vi "_Update Parameter Data.vi"(4 "error in":errorcluster, 7 "Parameter":T1 {"Expt"."Mass Range"."Resolution Type" items=["High/High", "Medium/Medium", "Low/Low", "High/Medium", "High/Low", "Medium/High", "Medium/Low", "Low/High", "Low/Medium"]}) -> (0 "error out":errorcluster, 1 "Last memory index":u16, 3 "RF Only":bool)   [LabVIEW 2015]
uses:
  Type/_RT Parameter.ctl
  Type/_RT Active Ch.ctl
  Type/_RT Expt.ctl
  Type/_Run Mode.ctl
  Type/_RT Mass Range.ctl
  Type/_RT Res Type.ctl
  _RT Global.vi
  <vilib>/Utility/error.llb/Error Cluster From Error Code.vi
  <vilib>/rvi/errors/niLvFpgaAdjustHostInterfaceError.vi
  <vilib>/rvi/interface/nirviReadWriteControl/nirviReadWriteControl.xnode
  Type/FPGA Typedef.ctl
  FPGA Bitfiles/FPGA9607.lvbitx
  NiFpgaLv.dll
panel:
  out "x-y":u32
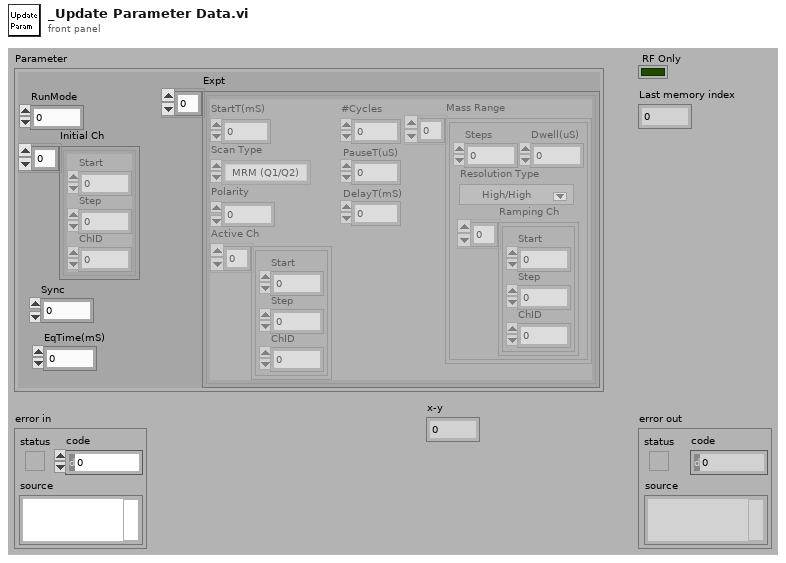
[diagram p1: front panel]
types:
  T1 = typedef "_RT Parameter.ctl" = cluster{"RunMode":i32, "Initial Ch":T2[], "Sync":u8, "Expt":T3[], "EqTime(mS)":i32}
  T2 = typedef "_RT Active Ch.ctl" = cluster{"Start":i32, "Step":i32, "ChID":i32}
  T3 = typedef "_RT Expt.ctl" = cluster{"StartT(mS)":i32, "#Cycles":i32, "Scan Type":T4, "PauseT(uS)":i32, "Polarity":u8, "DelayT(mS)":i32, "Active Ch":T2[], "Mass Range":T5[]}
  T4 = typedef "_Run Mode.ctl" = enum16{"MRM (Q1/Q2)", "Q1 Scan", "Q1 SRM", "Q2 Scan", "Q2 SRM", "Product Scan", "Precursor Scan", "Neutral Loss", "Neutral Gain"}
  T5 = typedef "_RT Mass Range.ctl" = cluster{"Steps":i32, "Dwell(uS)":i32, "Resolution Type":T6, "Ramping Ch":T2[]}
  T6 = typedef "_RT Res Type.ctl" = u16
  T7 = typedef "FPGA Typedef.ctl" = refnum<k20>
  T8 = typedef "_RT Configuration 2.ctl" = cluster{"Name":string, "Ch#":u8, "Min":dbl, "Max":dbl, "Def+":dbl, "Def-":dbl, "Offset":dbl, "Slope":dbl, "Type":u8, "Description":string, "SettleT":dbl}
  T9 = typedef "_RT Instrument 2.ctl" = cluster{"Table":T8[], "Instrument":string[]}
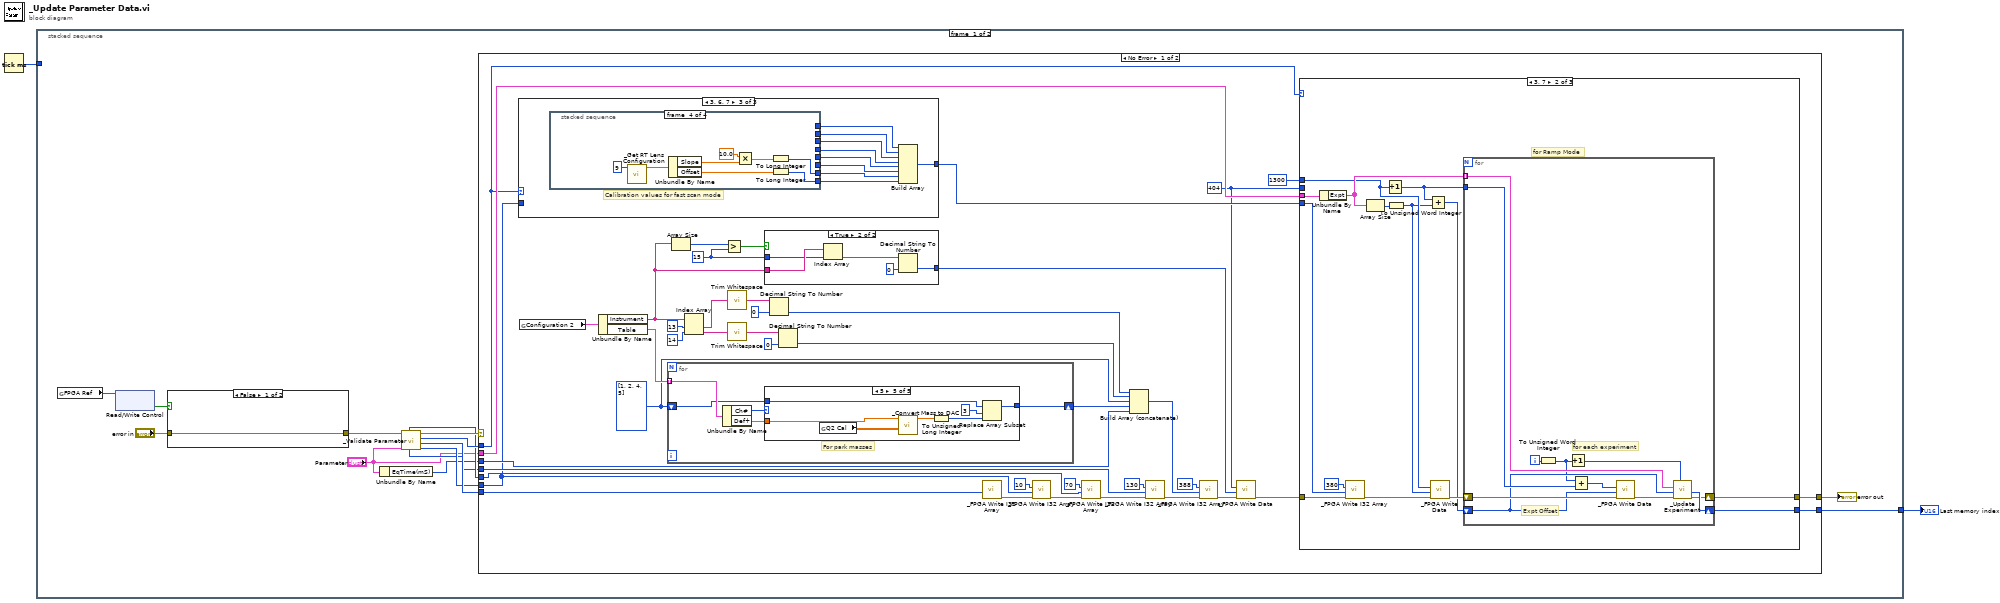
[diagram p0: block diagram]
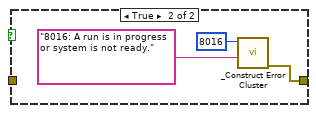
[diagram p2: hidden frame]
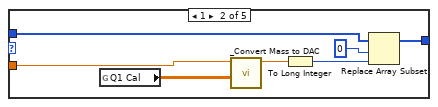
[diagram p5: hidden frame]
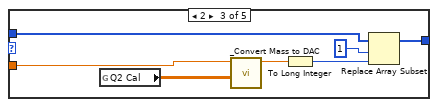
[diagram p6: hidden frame]
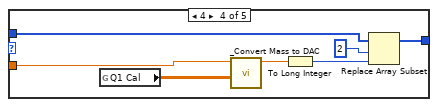
[diagram p7: hidden frame]
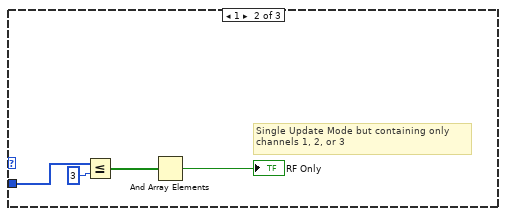
[diagram p9: hidden frame]
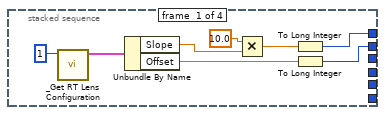
[diagram p10: hidden frame]
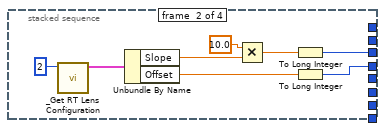
[diagram p11: hidden frame]
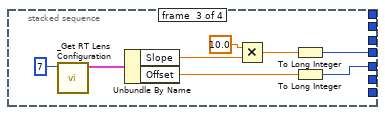
[diagram p12: hidden frame]
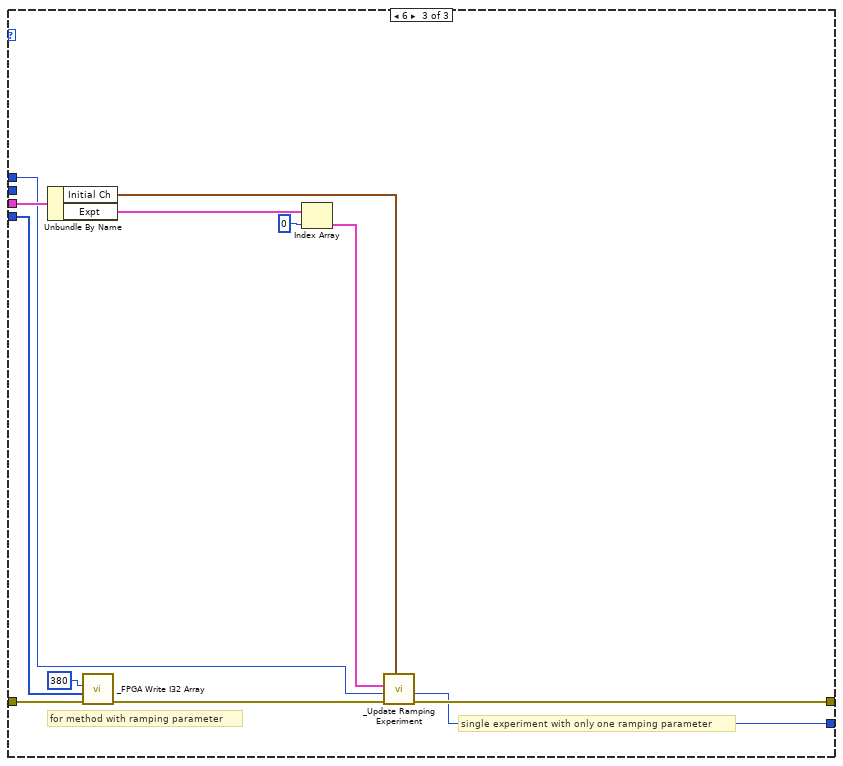
[diagram p14: hidden frame]
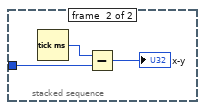
[diagram p16: hidden frame]
diagram:
  n1 = Tick Count (ms)() -> (millisecond timer value=w2:u32)
  n2 = stacked-sequence {
    tunnel: w2 -> [_ w189]
    tunnel: [w3 _] -> w1
    frame #0 {
      n3 = global read "_RT Global.vi" "FPGA Ref"() -> (w4:T7)
      n4 = xnode "Read/Write Control"("FPGA VI Reference In"=w4) -> ("Running"=w7:bool)  [unwired: 1 in, 2 out]
      n5 = case shown="False" w7 {
        tunnel: [w17 w18] -> w6
        tunnel: "error in" -> [w17 _]
        frame False {
        }
        frame True {
          n6 = call "_Construct Error Cluster.vi"("reason"="8016: A run is in progress or system is not ready.", "errorCode"=8016) -> ("error out"=w18:errorcluster)  [unwired: 2 in, 3 out]
        }
      }
      n7 = Unbundle By Name("Parameter") -> ("EqTime(mS)"=w8:i32)
      n8 = call "_Validate Parameter.vi"("Parameter"="Parameter", "error in (no error)"=w6) -> ("Ch ID"=w12:i32[], "General Param"=w13:i32[], "RunMode"=w14:i32, "error out"=w15:errorcluster, "Low Values"=w10:i32[], "High Values (DAC)"=w11:i32[])  [unwired: 2 out]
      n9 = case shown="No Error" w15 {
        selector: w15 -> [_ w187]
        tunnel: [w62 w187] -> w16
        tunnel: w14 -> [w50 _]
        tunnel: w13 -> [w60 _]
        tunnel: w12 -> [w31 _]
        tunnel: w11 -> [w55 _]
        tunnel: w10 -> [w53 _]
        tunnel: "Parameter" -> [w61 _]
        tunnel: w8 -> [w34 _]
        tunnel: [w23 _] -> w3
        frame No Error {
          w25 = 15 ("y")
          w22 = u16 404 ("y")
          w36 = u32[] [1, 2, 4, 5]
          n10 = case shown="3, 6, 7" w50 {
            tunnel: [_ _ w107] -> w49
            tunnel: w31 -> [_ w106 _]
            frame 0, Default {
            }
            frame 1 {
              # "Single Update Mode but containing only\nchannels 1, 2, or 3"
              n11 = Less Or Equal?(x=w106, y=3) -> (x <= y?=w104:bool[])
              n12 = And Array Elements(Boolean array=w104) -> (logical AND=→"RF Only":bool)
            }
            frame 3, 6, 7 {
              # "Calibration values for fast scan mode"
              n13 = stacked-sequence {
                tunnel: [w117 _ _ _] -> w108
                tunnel: [w116 _ _ _] -> w109
                tunnel: [_ w125 _ _] -> w110
                tunnel: [_ w124 _ _] -> w111
                tunnel: [_ _ w133 _] -> w112
                tunnel: [_ _ w132 _] -> w113
                tunnel: [_ _ _ w141] -> w114
                tunnel: [_ _ _ w140] -> w115
                frame #0 {
                  n14 = call "_Get RT Lens Configuration.vi"("Channel #"=u8 1) -> ("Lens Configuration"=w122:T8)  [unwired: 1 in, 5 out]
                  n15 = Unbundle By Name(w122) -> ("Slope"=w120:dbl, "Offset"=w121:dbl)
                  n16 = Multiply(x=10.0, y=w120) -> (x*y=w118:dbl)
                  n17 = To Long Integer(number=w118) -> (32bit integer=w117:i32)
                  n18 = To Long Integer(number=w121) -> (32bit integer=w116:i32)
                }
                frame #1 {
                  n19 = call "_Get RT Lens Configuration.vi"("Channel #"=u8 2) -> ("Lens Configuration"=w130:T8)  [unwired: 1 in, 5 out]
                  n20 = Unbundle By Name(w130) -> ("Slope"=w128:dbl, "Offset"=w129:dbl)
                  n21 = Multiply(x=10.0, y=w128) -> (x*y=w126:dbl)
                  n22 = To Long Integer(number=w126) -> (32bit integer=w125:i32)
                  n23 = To Long Integer(number=w129) -> (32bit integer=w124:i32)
                }
                frame #2 {
                  n24 = call "_Get RT Lens Configuration.vi"("Channel #"=u8 7) -> ("Lens Configuration"=w138:T8)  [unwired: 1 in, 5 out]
                  n25 = Unbundle By Name(w138) -> ("Slope"=w136:dbl, "Offset"=w137:dbl)
                  n26 = Multiply(x=10.0, y=w136) -> (x*y=w134:dbl)
                  n27 = To Long Integer(number=w134) -> (32bit integer=w133:i32)
                  n28 = To Long Integer(number=w137) -> (32bit integer=w132:i32)
                }
                frame #3 {
                  n29 = call "_Get RT Lens Configuration.vi"("Channel #"=u8 9) -> ("Lens Configuration"=w146:T8)  [unwired: 1 in, 5 out]
                  n30 = Unbundle By Name(w146) -> ("Slope"=w144:dbl, "Offset"=w145:dbl)
                  n31 = Multiply(x=10.0, y=w144) -> (x*y=w142:dbl)
                  n32 = To Long Integer(number=w142) -> (32bit integer=w141:i32)
                  n33 = To Long Integer(number=w145) -> (32bit integer=w140:i32)
                }
              }
              n34 = Build Array(w108, w109, w110, w111, w112, w113, w114, w115) -> (w107:i32[])
            }
          }
          n35 = global read "_RT Global.vi" "Configuration 2"() -> (w48:T9)
          n36 = Unbundle By Name(w48) -> ("Instrument"=w26:string[], "Table"=w41:T8[])
          n37 = for {
            tunnel: w41 -> [w73] mode=indexing
            shift-right: [w70] -> w35
            shift-left: w36 -> [w71]
            # "For park masses"
            n38 = Unbundle By Name(w73) -> ("Ch#"=w72:u8, "Def+"=w69:dbl)
            n39 = case shown="5" w72 {
              tunnel: w71 -> [w74 w78 w85 w92 w99]
              tunnel: [w74 w75 w82 w89 w96] -> w70
              tunnel: w69 -> [_ w81 w88 w95 w102]
              frame 0, Default {
              }
              frame 1 {
                n40 = global read "_RT Global.vi" "Q1 Cal"() -> (w80:dbl[][])
                n41 = call "_Convert Mass to DAC.vi"("Calibration Table"=w80, "Mass"=w81) -> ("DAC Value"=w79:dbl)  [unwired: 2 in, 3 out]
                n42 = To Long Integer(number=w79) -> (32bit integer=w76:i32)
                n43 = Replace Array Subset(array=w78, new element=w76, index=0) -> (w75:u32[])
              }
              frame 2 {
                n44 = global read "_RT Global.vi" "Q2 Cal"() -> (w87:dbl[][])
                n45 = call "_Convert Mass to DAC.vi"("Calibration Table"=w87, "Mass"=w88) -> ("DAC Value"=w86:dbl)  [unwired: 2 in, 3 out]
                n46 = To Long Integer(number=w86) -> (32bit integer=w83:i32)
                n47 = Replace Array Subset(array=w85, new element=w83, index=1) -> (w82:u32[])
              }
              frame 4 {
                n48 = global read "_RT Global.vi" "Q1 Cal"() -> (w94:dbl[][])
                n49 = call "_Convert Mass to DAC.vi"("Calibration Table"=w94, "Mass"=w95) -> ("DAC Value"=w93:dbl)  [unwired: 2 in, 3 out]
                n50 = To Long Integer(number=w93) -> (32bit integer=w90:i32)
                n51 = Replace Array Subset(array=w92, new element=w90, index=2) -> (w89:u32[])
              }
              frame 5 {
                n52 = global read "_RT Global.vi" "Q2 Cal"() -> (w101:dbl[][])
                n53 = call "_Convert Mass to DAC.vi"("Calibration Table"=w101, "Mass"=w102) -> ("DAC Value"=w100:dbl)  [unwired: 2 in, 3 out]
                n54 = To Unsigned Long Integer(number=w100) -> (unsigned 32bit integer=w97:u32)
                n55 = Replace Array Subset(array=w99, new element=w97, index=3) -> (w96:u32[])
              }
            }
          }
          n56 = Array Size(array=w26) -> (size(s)=w28:i32)
          n57 = Index Array(array=w26, index #1=13 ("index"), index #2=14 ("index")) -> (element #1=w45:string, element #2=w44:string)
          n58 = Greater?(x=w28, y=w25) -> (0:w27:bool)
          n59 = call <vilib>:"Trim Whitespace.vi"("string"=w45) -> ("trimmed string"=w33:string)  [unwired: 1 in]
          n60 = call <vilib>:"Trim Whitespace.vi"("string"=w44) -> ("trimmed string"=w43:string)  [unwired: 1 in]
          n61 = case shown="True" w27 {
            tunnel: w26 -> [_ w68]
            tunnel: w25 -> [w63 w66]
            tunnel: [w63 w65] -> w24
            frame False {
            }
            frame True {
              n62 = Index Array(array=w68, index=w66) -> (element=w67:string)
              n63 = Decimal String To Number(string=w67, default (0L)=u32 0 ("default (0 I32)")) -> (number=w65:u32)  [unwired: 2 out]
            }
          }
          n64 = Decimal String To Number(string=w33, default (0L)=u32 0 ("default (0 I32)")) -> (number=w32:u32)  [unwired: 2 out]
          n65 = Decimal String To Number(string=w43, default (0L)=u32 0 ("default (0 I32)")) -> (number=w40:u32)  [unwired: 2 out]
          n66 = call "_FPGA Write I32 Array.vi"("U32 Array"=w60) -> ("error out"=w58:errorcluster)  [unwired: 4 in, 2 out]
          n67 = call "_FPGA Write I32 Array.vi"("error in"=w58, "U32 Array"=w31, "Offset (0)"=u16 10 ("y")) -> ("error out"=w56:errorcluster)  [unwired: 2 in, 2 out]
          n68 = call "_FPGA Write I32 Array.vi"("error in"=w56, "U32 Array"=w55, "Offset (0)"=u16 70 ("y")) -> ("error out"=w52:errorcluster)  [unwired: 2 in, 2 out]
          n69 = Build Array (concatenate)(w32, w40, w36, w35, w34) -> (w37:u32[])
          n70 = call "_FPGA Write I32 Array.vi"("error in"=w52, "U32 Array"=w53, "Offset (0)"=u16 130 ("y")) -> ("error out"=w39:errorcluster)  [unwired: 2 in, 2 out]
          n71 = call "_FPGA Write I32 Array.vi"("error in"=w39, "U32 Array"=w37, "Offset (0)"=u16 388 ("y")) -> ("error out"=w30:errorcluster)  [unwired: 2 in, 2 out]
          n72 = call "_FPGA Write Data.vi"("error in"=w30, "Data"=w24, "Address"=w22) -> ("error out"=w29:errorcluster)  [unwired: 5 in]
          n73 = case shown="3, 7" w50 {
            tunnel: [w149 w159 w183] -> w62
            tunnel: w61 -> [_ w158 w186]
            tunnel: w29 -> [w149 w154 w178]
            tunnel: u16 1300 ("Address") -> [_ w156 w181]
            tunnel: w49 -> [_ w152 w176]
            tunnel: [w148 w151 w175] -> w23
            tunnel: w22 -> [w148 _ _]
            frame Default {
            }
            frame 3, 7 {
              # "for Ramp Mode"
              n74 = Unbundle By Name(w158) -> ("Expt"=w163:T3[])
              n75 = call "_FPGA Write I32 Array.vi"("error in"=w154, "U32 Array"=w152, "Offset (0)"=u16 380 ("y")) -> ("error out"=w153:errorcluster)  [unwired: 2 in, 2 out]
              n76 = Array Size(array=w163) -> (size(s)=w157:i32)
              n77 = Increment(x=w156) -> (x+1=w160:u16)
              n78 = To Unsigned Word Integer(number=w157) -> (unsigned 16bit integer=w150:u16)
              n79 = Add(x=w160, y=w150) -> (x+y=w161:u16)
              n80 = call "_FPGA Write Data.vi"("error in"=w153, "Data"=w150, "Address"=w156) -> ("error out"=w162:errorcluster)  [unwired: 3 in, 2 out]
              n81 = for {
                tunnel: w163 -> [w172] mode=indexing
                shift-right: [w167] -> w159
                shift-left: w162 -> [w174]
                tunnel: w160 -> [w173]
                shift-right: [w168] -> w151
                shift-left: w161 -> [w169]
                i -> [w166]
                # "for each experiment"
                # "Expt Offset"
                n82 = To Unsigned Word Integer(number=w166) -> (unsigned 16bit integer=w164:u16)
                n83 = Increment(x=w164) -> (x+1=w165:u16)
                n84 = Add(x=w164, y=w173) -> (x+y=w170:u16)
                n85 = call "_FPGA Write Data.vi"("error in"=w174, "Data"=w169, "Address"=w170) -> ("error out"=w171:errorcluster)  [unwired: 3 in, 2 out]
                n86 = call "_Update Experiment.vi"("Expt#"=w165, "error in"=w171, "Offset"=w169, "Expt"=w172) -> ("error out"=w167:errorcluster, "Next Offset"=w168:u16)  [unwired: 1 in, 2 out]
              }
            }
            frame 6 {
              # "single experiment with only one ramping parameter"
              # "for method with ramping parameter"
              n87 = Unbundle By Name(w186) -> ("Initial Ch"=w180:T2[], "Expt"=w185:T3[])
              n88 = call "_FPGA Write I32 Array.vi"("error in"=w178, "U32 Array"=w176, "Offset (0)"=380 ("y")) -> ("error out"=w177:errorcluster)  [unwired: 2 in, 2 out]
              n89 = Index Array(array=w185, index=0) -> (element=w182:T3)
              n90 = call "_Update Ramping Experiment.vi"("Ramping Ch"=w180, "error in"=w177, "Offset"=w181, "Expt"=w182) -> ("error out"=w183:errorcluster, "Next Offset"=w175:u16)  [unwired: 1 in, 2 out]
            }
          }
        }
        frame Error {
        }
      }
      "error out" <- w16
    }
    frame #1 {
      n91 = Tick Count (ms)() -> (millisecond timer value=w190:u32)
      n92 = Subtract(x=w190, y=w189) -> (x-y=→"x-y":u32)
    }
  }
  "Last memory index" <- w1
